vi "Connection Manager (customizable TDT).vi"(9 "Required":cluster{"DI":string[]}[](array[cluster]), 11 "Configuration file":path=path "C:/ProgramData/EPL/Tosca Defaults.ini") -> (2 "changed?":bool)   [LabVIEW 2020]
uses:
  Utility VIs/Controls/KTable/KTable.xctl
  Utility VIs/Controls/KListboxEx/KListboxEx.xctl
  PXI DAQ VIs/TDT VIs/Typedefs/TDT-Input source.ctl
  Type Defs/CM-Connection.ctl
  Utility VIs/Controls/KTable/Event Type.ctl
  PXI DAQ VIs/TDT VIs/TDT-Globals.vi
panel:
  in  "AI List":i32(xcontrol) caption="Inputs"
  in  "DI List":i32(xcontrol) caption="Inputs"
  in  "AO List":i32(xcontrol) caption="Outputs"
  in  "DO List":i32(xcontrol) caption="Outputs"
  in  "Apply Button":bool
  out "Save Op":enum16{"None", "Save", "Save and Exit"}(ring)
  in  "Exit":bool
  in  "DO Table":u16(xcontrol)
  out "show device":bool
  out "Image":enum32{"Blank", "RX6", "RZ5", "RZ6"}(tab)
  in  "Input source":u16(ring) items=["Front panel", "RA4LI", "RA16LI"]
  in  "Run on":i16(ring) items=[""=-1, "RX6"=0, "RZ5"=1, "RZ6"=2]
  in  "DI Table":u16(xcontrol)
  in  "AI Table":u16(xcontrol)
  out "read config":bool
  out "show connections":bool
  in  "AO Table":u16(xcontrol)
  # "ANALOG"
  # "DIGITAL"
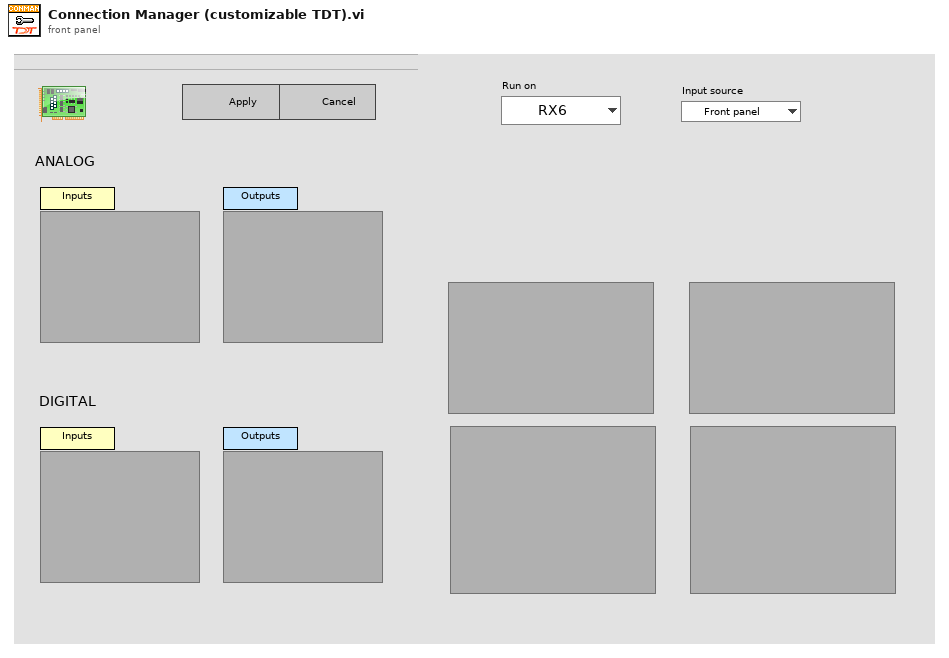
[diagram p1: front panel]
types:
  T1 = typedef "KListboxEx.xctl/Events.ctl" = cluster{"Items Changed":refnum<user-event>, "List Changed":refnum<user-event>}
  T2 = typedef "KTable.xctl/Events.ctl" = cluster{"Items Changed":refnum<user-event>}
  T3 = typedef "TDT-Input source.ctl" = enum16{"Front Panel", "RA4LI", "RA16LI"}
  T4 = typedef "KTable.xctl/Event Type.ctl" = enum16{"None", "Selection", "Edit", "Insert", "Delete", "Up", "Down", "Duplicate"}
  T5 = typedef "TDT-Output source.ctl" = cluster{"Device":T6, "Num":i32}
  T6 = typedef "TDT-Device ID.ctl" = enum16{"None", "PA5", "RP2", "RL2", "RA16", "RV8", "RX5", "RX6", "RX7", "RX8", "RZ2", "RZ5", "RZ6"}
  T7 = typedef "TDT-Device Config.ctl" = cluster{"Output":T5, "Input":T3}
  T8 = typedef "CM-Connection.ctl" = cluster{"IOChannel":string, "Endpoint":string}
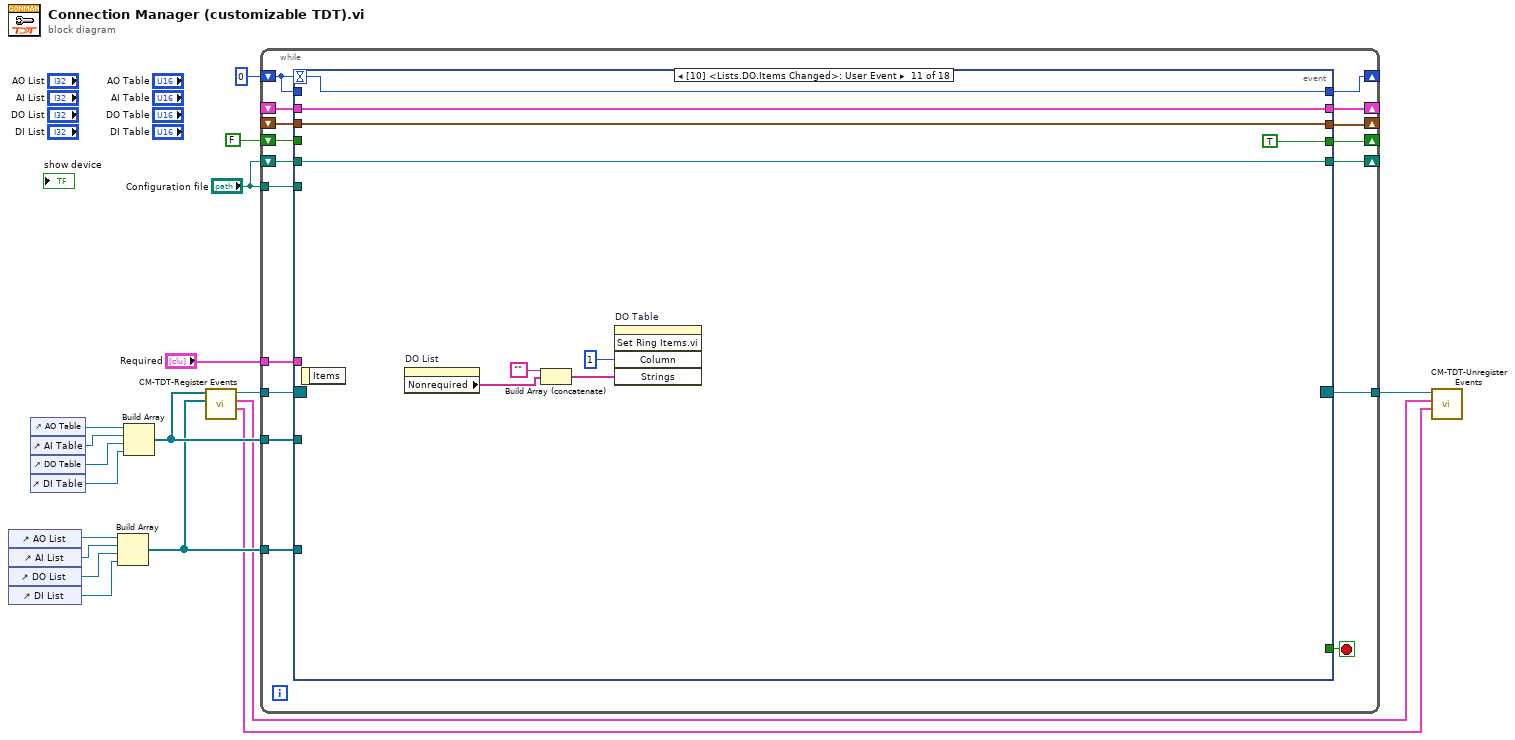
[diagram p0: block diagram]
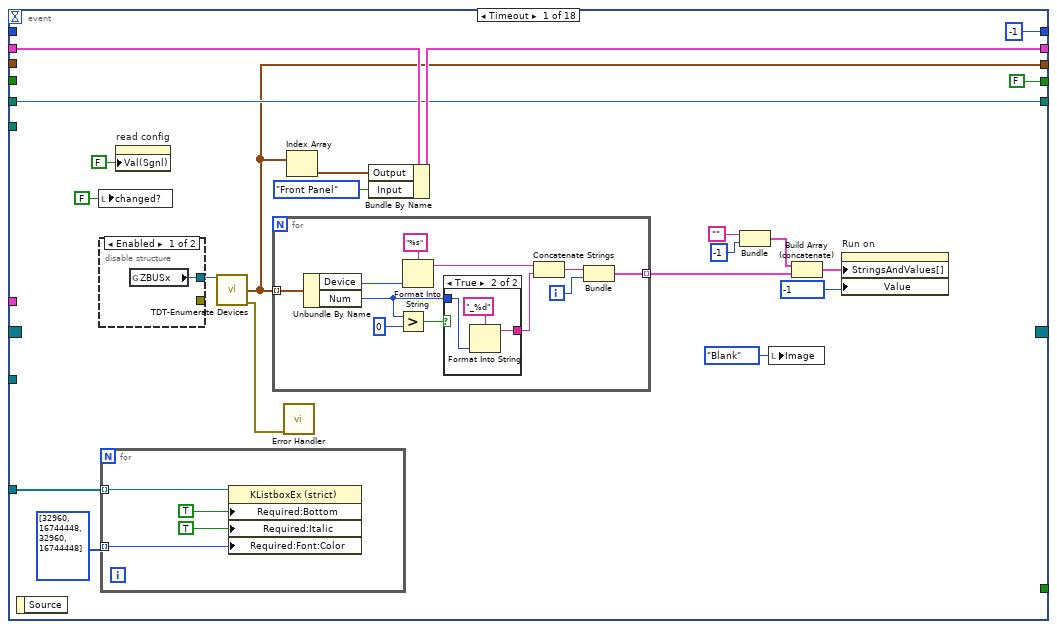
[diagram p2: hidden frame]
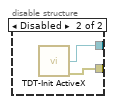
[diagram p3: hidden frame]
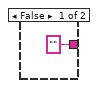
[diagram p4: hidden frame]
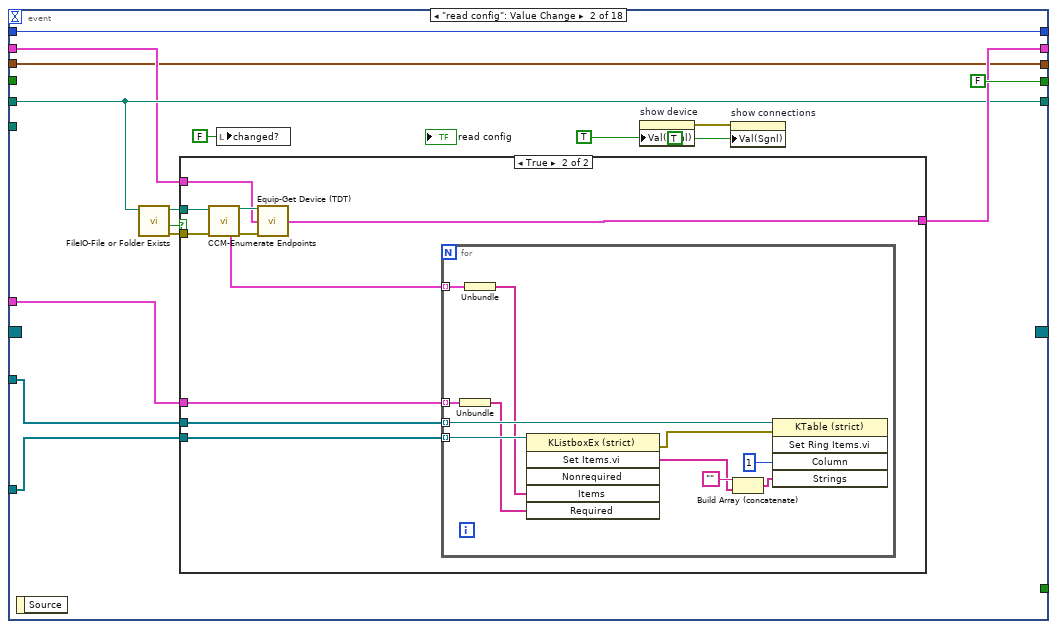
[diagram p5: hidden frame]
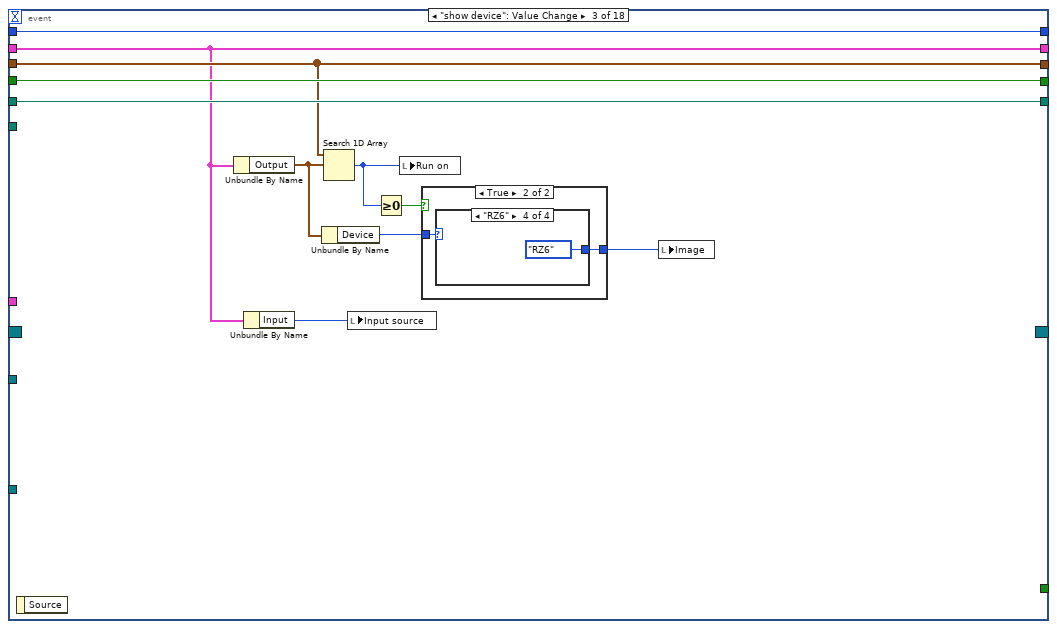
[diagram p7: hidden frame]
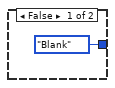
[diagram p8: hidden frame]
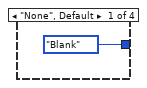
[diagram p9: hidden frame]
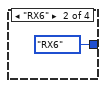
[diagram p10: hidden frame]
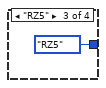
[diagram p11: hidden frame]
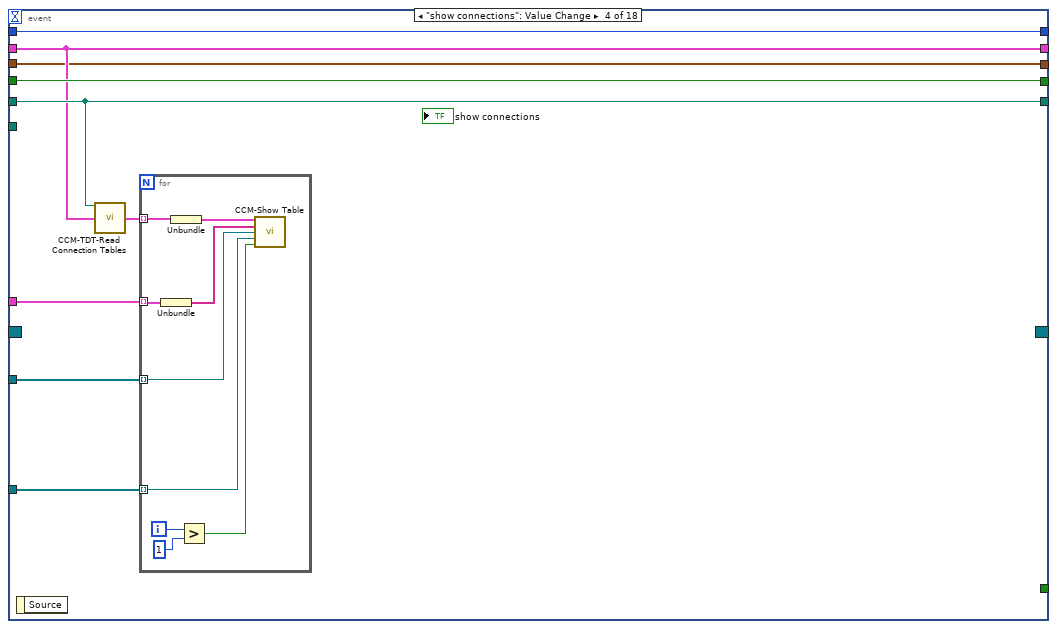
[diagram p12: hidden frame]
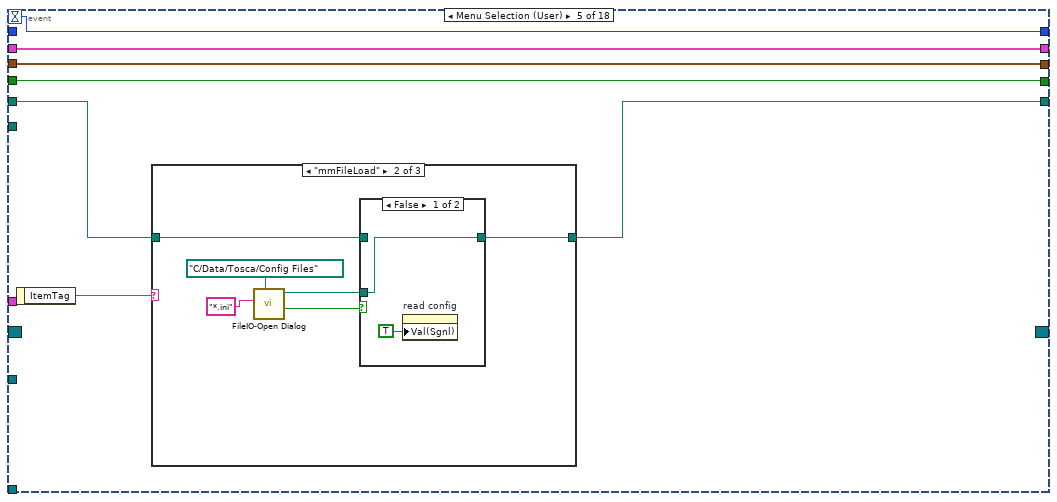
[diagram p13: hidden frame]
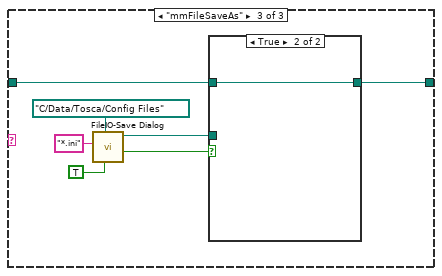
[diagram p16: hidden frame]
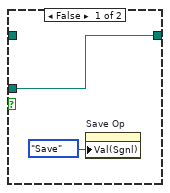
[diagram p17: hidden frame]
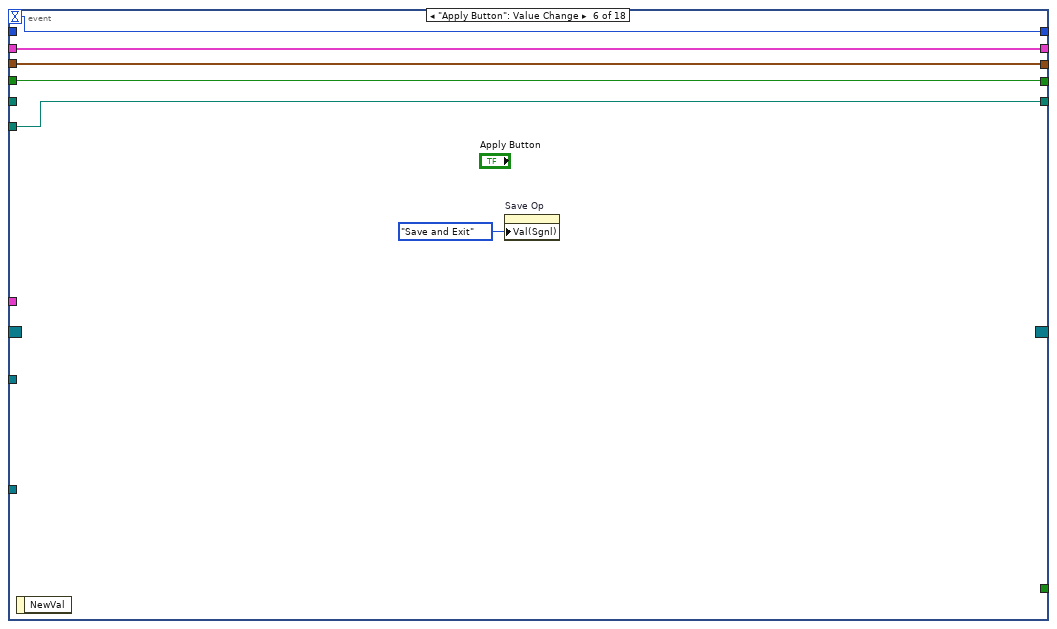
[diagram p18: hidden frame]
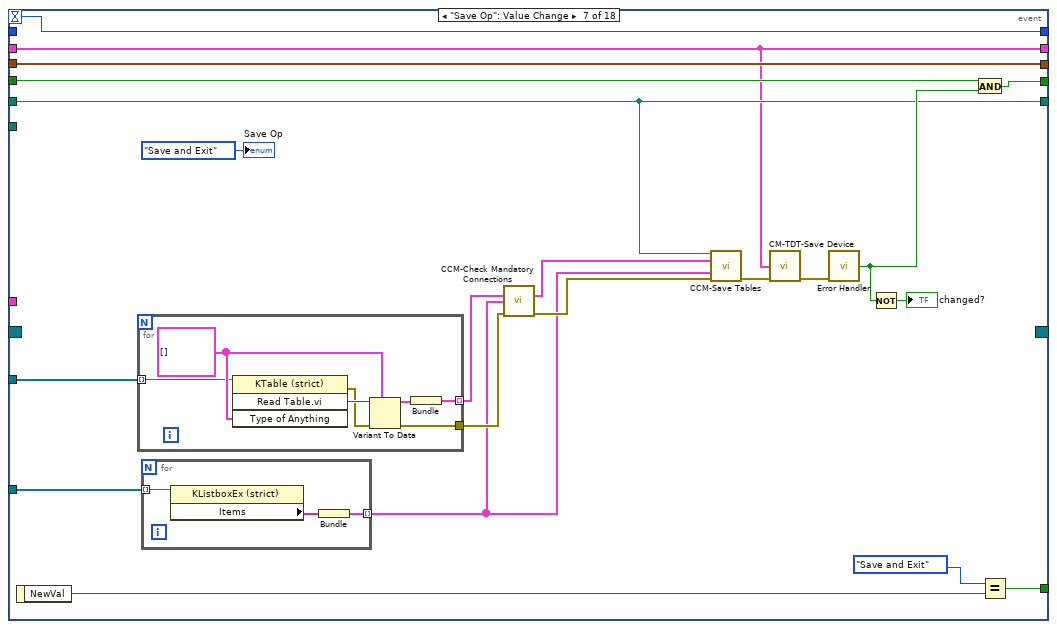
[diagram p19: hidden frame]
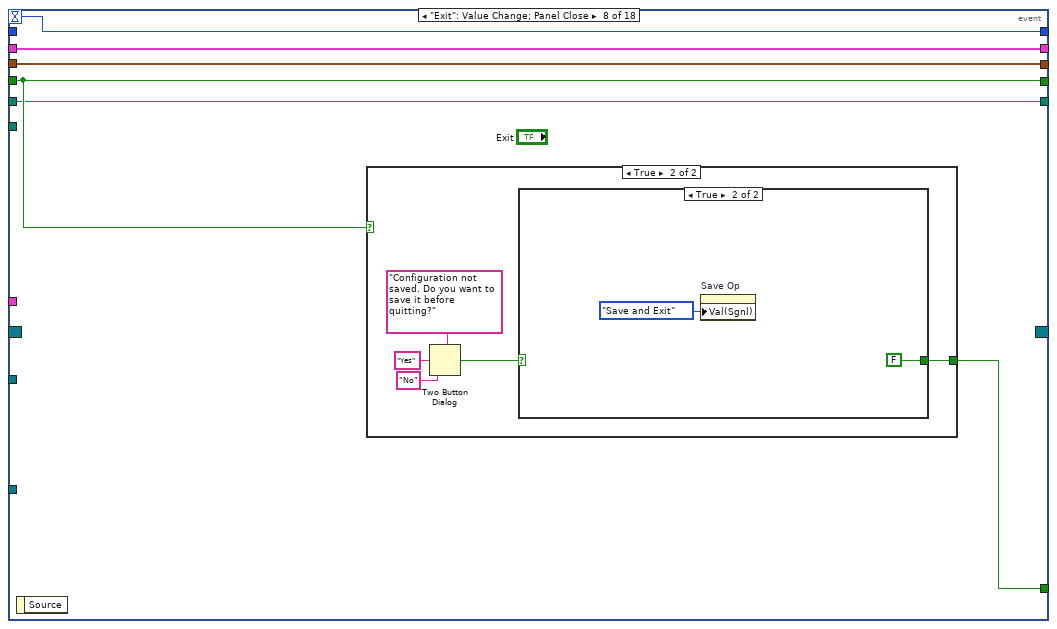
[diagram p20: hidden frame]
diagram:
  n1 = control-ref of="AO List"() -> (w6:refnum<vi>)
  n2 = control-ref of="AI List"() -> (w11:refnum<vi>)
  n3 = control-ref of="DO List"() -> (w10:refnum<vi>)
  n4 = control-ref of="DI List"() -> (w5:refnum<vi>)
  n5 = control-ref of="AO Table"() -> (w14:refnum<vi>)
  n6 = control-ref of="AI Table"() -> (w13:refnum<vi>)
  n7 = control-ref of="DO Table"() -> (w9:refnum<vi>)
  n8 = control-ref of="DI Table"() -> (w12:refnum<vi>)
  n9 = Build Array(w6, w11, w10, w5) -> (w7:refnum<vi>[])
  n10 = Build Array(w14, w13, w9, w12) -> (w8:refnum<vi>[])
  n11 = call "CM-TDT-Register Events.vi"("List Refs"=w7, "Table Refs"=w8) -> ("Lists"=w2:cluster{"AO":T1, "AI":T1, "DO":T1, "DI":T1}, "Tables"=w3:cluster{"AO":T2, "AI":T2, "DO":T2, "DI":T2}, "Event Registration Refnum"=w16:refnum<event-registration>)  [unwired: 7 in]
  n12 = while {
    shift-right: [w34] -> _
    shift-left: 0 -> [w29]
    shift-right: [w31] -> _
    shift-left: FALSE -> [w32]
    tunnel: "Required" -> [w30]
    tunnel: w16 -> [w28]
    shift-right: [w27] -> _
    shift-left: _ -> [w26]
    shift-right: [w25] -> _
    shift-left: "Configuration file" -> [w33]
    tunnel: "Configuration file" -> [w24]
    tunnel: w8 -> [w23]
    shift-right: [w22] -> _
    shift-left: _ -> [w21]
    tunnel: w7 -> [w20]
    tunnel: [w19] -> w4
    stop <- w35 stop-if-true
    n13 = event shown="[10] <Lists.DO.Items Changed>: User Event" {
      selector: w28 -> [_ _ _ _ _ _ _ _ _ _ _ _ _ _ _ _ _ _]
      dyn-events: [_ _ _ _ _ _ _ _ _ _ _ _ _ _ _ _ _ _] -> w19
      timeout: w29 -> [_ _ _ _ w159 w184 w206 w222 w240 w249 w258 w267 _ _ _ _ _ _]
      tunnel: [_ _ _ _ _ _ w202 w221 _ _ _ _ _ _ _ _ _ _] -> w35
      tunnel: [-1 w89 w127 w142 w159 w184 w206 w222 w240 w249 w258 w267 w278 w290 w299 w308 w317 w326] -> w34
      tunnel: w33 -> [w49 w87 w125 w141 w155 _ w197 w218 w238 w247 w256 w265 w276 w288 w297 w306 w315 w324]
      tunnel: w32 -> [_ _ w126 w143 w158 w183 w201 w220 _ _ _ _ _ _ w293 w302 w311 w320]
      tunnel: [FALSE FALSE w126 w143 w158 w183 w200 w220 TRUE TRUE TRUE TRUE TRUE TRUE w292 w301 w310 w319] -> w31
      tunnel: w30 -> [_ w79 _ w136 _ _ _ _ _ _ _ _ _ _ _ _ _ _]
      tunnel: w29 -> [_ w89 w127 w142 _ _ _ _ _ _ _ _ w278 w290 w299 w308 w317 w326]
      tunnel: [w51 w88 w121 w140 w156 w182 w189 w219 w239 w248 w257 w266 w275 w286 w298 w307 w316 w325] -> w27
      tunnel: w26 -> [w52 w86 w121 w140 w156 w182 w189 w219 w239 w248 w257 w266 w277 w289 w298 w307 w316 w325]
      tunnel: [w49 w87 w125 w141 w154 w181 w197 w218 w238 w247 w256 w265 w276 w288 w297 w306 w315 w324] -> w25
      tunnel: w24 -> [_ _ _ _ _ w181 _ _ _ _ _ _ _ _ _ _ _ _]
      tunnel: w23 -> [_ w85 _ w137 _ _ w194 _ _ _ _ _ _ _ _ _ _ _]
      tunnel: [w47 w84 w124 w139 w153 w180 w195 w217 w237 w246 w255 w264 w274 w287 w296 w305 w314 w323] -> w22
      tunnel: w21 -> [_ w84 w124 w139 w153 w180 w195 w217 w237 w246 w255 w264 w274 w287 w296 w305 w314 w323]
      tunnel: w20 -> [w37 w80 _ w135 _ _ w192 _ _ _ _ _ _ _ _ _ _ _]
      event Timeout {
        w40 = i16 -1 items=["", "RZ5_1"] ("Run on")
        n14 = event-data() -> ()  [unwired: 1 in, 1 out]
        n15 = local write "changed?"(FALSE ("changed?")) -> ()
        n16 = disable-structure shown="Enabled" {
          disable-tunnel: [w61 w63] -> w53
          disable-tunnel: [_ w62] -> _
          frame Enabled {
            n17 = global read "TDT-Globals.vi" "ZBUSx"() -> (w61:refnum<k7>)
          }
          frame Disabled {
            n18 = call "TDT-Init ActiveX.vi"() -> ("ZBUSx"=w63:refnum<k7>, "error out"=w62:errorcluster)  [unwired: 12 in, 2 out]
          }
        }
        n19 = for {
          tunnel: w37 -> [w58] mode=indexing
          tunnel: u32[] [32960, 16744448, 32960, 16744448] -> [w57] mode=indexing
          n20 = property class="KListboxEx (strict)"(reference=w58, "Required:Bottom"=TRUE, "Required:Italic"=TRUE ("Required:Font:Italic"), "Required:Font:Color"=w57) -> ()  [unwired: 1 in, 2 out]
        }
        n21 = property on="read config" class="Bool (strict)"("Val(Sgnl)"=FALSE ("Value (Signaling)")) -> ()  [unwired: 2 in, 2 out]
        n22 = call "TDT-Enumerate Devices.vi"("ZBUSx In"=w53) -> ("Devices"=w47:T5[], "error out"=w38:errorcluster)  [unwired: 12 in, 1 out]
        n23 = for {
          tunnel: w47 -> [w74] mode=indexing
          tunnel: [w65] -> w42 mode=indexing
          i -> [w64]
          n24 = Unbundle By Name(w74) -> ("Device"=w66:T6, "Num"=w69:i32)
          n25 = Greater?(x=w69, y=0) -> (0:w70:bool)
          n26 = Format Into String(format string="%s", w66) -> (resulting string=w72:string)  [unwired: 2 in, 1 out]
          n27 = case shown="True" w70 {
            tunnel: w69 -> [_ w77]
            tunnel: ["" w76] -> w67
            frame False {
            }
            frame True {
              n28 = Format Into String(format string="_%d", w77) -> (resulting string=w76:string)  [unwired: 2 in, 1 out]
            }
          }
          n29 = Concatenate Strings(w72, w67) -> (w68:string)
          n30 = Bundle(w68, w64) -> (w65:cluster{string, i32})  [unwired: 1 in]
        }
        n31 = call "Error Handler.vi"("error in (no error)"=w38) -> ()  [unwired: 13 in, 2 out]
        n32 = Index Array(array=w47) -> (element=w50:T5)  [unwired: 1 in]
        n33 = Bundle By Name(cluster=w52, "Output"=w50, "Input"=TDT-Input_source."Front Panel") -> (w51:T7)
        n34 = Bundle("", -1) -> (w41:cluster{string, i32})  [unwired: 1 in]
        n35 = local write "Image"(enum32{"Blank", "RX6", "RZ5"}."Blank" ("Image")) -> ()
        n36 = Build Array (concatenate)(w41, w42) -> (w43:cluster{string, i32}[])
        n37 = property on="Run on" class="Ring (strict)"("StringsAndValues[]"=w43, "Value"=w40) -> ()  [unwired: 2 in, 2 out]
      }
      event "read config": Value Change {
        n38 = event-data() -> ()  [unwired: 1 in, 1 out]
        n39 = call "FileIO-File or Folder Exists.vi"("path"=w87) -> ("error out"=w93:errorcluster, "Exists?"=w92:bool, "dup path"=w94:path)  [unwired: 7 in, 1 out]
        n40 = case shown="True" w92 {
          tunnel: w94 -> [_ w105]
          tunnel: w93 -> [_ w104]
          tunnel: [w95 w100] -> w88
          tunnel: w86 -> [w95 w101]
          tunnel: w85 -> [_ w99]
          tunnel: w80 -> [_ w98]
          tunnel: w79 -> [_ w97]
          frame False {
          }
          frame True {
            n41 = call "CCM-Enumerate Endpoints.vi"("Path In"=w105, "error in (no error)"=w104) -> ("Path Out"=w102:path, "Endpoints"=w96:cluster{"Name":string[]}[], "error out"=w103:errorcluster)  [unwired: 9 in, 2 out]
            n42 = call "Equip-Get Device (TDT).vi"("Path In"=w102, "Default"=w101, "error in (no error)"=w103) -> ("TDT-Device Config"=w100:T7)  [unwired: 10 in, 2 out]
            n43 = for {
              tunnel: w99 -> [w113] mode=indexing
              tunnel: w98 -> [w112] mode=indexing
              tunnel: w96 -> [w110] mode=indexing
              tunnel: w97 -> [w109] mode=indexing
              n44 = Unbundle(w109) -> ("DI"=w108:string[])
              n45 = Unbundle(w110) -> ("Name"=w107:string[])
              n46 = invoke on="Invoke Node" class="KListboxEx (strict)" method="Set Items.vi"(reference=w112, "Items"=w107, "Required"=w108) -> (error out=w111:errorcluster, "Set Items.vi"=w106:string[])  [unwired: 3 in, 4 out]
              n47 = Build Array (concatenate)("", w106) -> (w115:string[])
              n48 = invoke on="Invoke Node" class="KTable (strict)" method="Set Ring Items.vi"(reference=w113, error in=w111, "Column"=1, "Strings"=w115) -> ()  [unwired: 1 in, 5 out]
            }
          }
        }
        n49 = local write "changed?"(FALSE ("changed?")) -> ()
        n50 = property on="show device" class="Bool (strict)"("Val(Sgnl)"=TRUE ("Value (Signaling)")) -> (error out=w82:errorcluster)  [unwired: 2 in, 1 out]
        n51 = property on="show connections" class="Bool (strict)"(error in=w82, "Val(Sgnl)"=TRUE ("Value (Signaling)")) -> ()  [unwired: 1 in, 2 out]
      }
      event "show device": Value Change {
        n52 = event-data() -> ()  [unwired: 1 in, 1 out]
        n53 = Unbundle By Name(w121) -> ("Output"=w122:T5)
        n54 = Unbundle By Name(w121) -> ("Input"=w120:T3)
        n55 = Unbundle By Name(w122) -> ("Device"=w123:T6)
        n56 = Search 1D Array(1D array=w124, element=w122) -> (index of element=w119:i32)  [unwired: 1 in]
        n57 = local write "Input source"(w120) -> ()
        n58 = Greater Or Equal To 0?(x=w119) -> (x >= 0?=w118:bool)
        n59 = local write "Run on"(w119) -> ()
        n60 = case shown="True" w118 {
          tunnel: w123 -> [_ w130]
          tunnel: [enum32{"Blank", "RX6", "RZ5"}."Blank" ("Image") w129] -> w117
          frame False {
          }
          frame True {
            n61 = case shown="\"RZ6\"" w130 {
              tunnel: [enum32{"Blank", "RX6", "RZ5"}."Blank" ("Image") enum32{"Blank", "RX6", "RZ5"}."RX6" ("Image") enum32{"Blank", "RX6", "RZ5"}."RZ5" ("Image") enum32{"Blank", "RX6", "RZ5", "RZ6"}."RZ6" ("Image")] -> w129
              frame "None", Default {
              }
              frame "RX6" {
              }
              frame "RZ5" {
              }
              frame "RZ6" {
              }
            }
          }
        }
        n62 = local write "Image"(w117) -> ()
      }
      event "show connections": Value Change {
        n63 = event-data() -> ()  [unwired: 1 in, 1 out]
        n64 = call "CCM-TDT-Read Connection Tables.vi"("Path In"=w141, "TDT-Device Config"=w140) -> ("Tables"=w138:cluster{"Table":T8[]}[])  [unwired: 12 in, 1 out]
        n65 = for {
          tunnel: w138 -> [w150] mode=indexing
          tunnel: w137 -> [w146] mode=indexing
          tunnel: w136 -> [w148] mode=indexing
          tunnel: w135 -> [w145] mode=indexing
          i -> [w152]
          n66 = Unbundle(w148) -> ("DI"=w147:string[])
          n67 = Unbundle(w150) -> ("Table"=w149:T8[])
          n68 = Greater?(x=w152, y=1) -> (0:w144:bool)
          n69 = call "CCM-Show Table.vi"("Table"=w149, "Required"=w147, "Table Ref"=w146, "List Ref"=w145, "Force required"=w144) -> ()  [unwired: 11 in]
        }
      }
      event Menu Selection (User) {
        n70 = event-data() -> ("ItemTag"=w157:string)  [unwired: 1 in]
        n71 = case shown="\"mmFileLoad\"" w157 {
          tunnel: w155 -> [w160 w162 w171]
          tunnel: [w160 w161 w170] -> w154
          frame "False", Default {
          }
          frame "mmFileLoad" {
            n72 = call "FileIO-Open Dialog.vi"("Default Folder"=path "C:/Data/Tosca/Config Files", "pattern (all files)"="*.ini") -> ("cancelled"=w164:bool, "selected path"=w163:path)  [unwired: 7 in, 1 out]
            n73 = case shown="False" w164 {
              tunnel: w163 -> [w168 _]
              tunnel: w162 -> [_ w169]
              tunnel: [w168 w169] -> w161
              frame False {
                n74 = property on="read config" class="Bool (strict)"("Val(Sgnl)"=TRUE ("Value (Signaling)")) -> ()  [unwired: 2 in, 2 out]
              }
              frame True {
              }
            }
          }
          frame "mmFileSaveAs" {
            n75 = call "FileIO-Save Dialog.vi"("Overwrite prompt?"=TRUE, "Default Folder"=path "C:/Data/Tosca/Config Files", "pattern (all files)"="*.ini") -> ("cancelled"=w173:bool, "selected path"=w172:path)  [unwired: 6 in, 1 out]
            n76 = case shown="True" w173 {
              tunnel: w172 -> [w177 _]
              tunnel: w171 -> [_ w179]
              tunnel: [w177 w179] -> w170
              frame False {
                n77 = property on="Save Op" class="Enum (strict)"("Val(Sgnl)"=enum16{"None", "Save", "Save and Exit"}."Save" ("Value (Signaling)")) -> ()  [unwired: 2 in, 2 out]
              }
              frame True {
              }
            }
          }
        }
      }
      event "Apply Button": Value Change {
        n78 = event-data() -> ()  [unwired: 1 in, 1 out]
        n79 = property on="Save Op" class="Enum (strict)"("Val(Sgnl)"=enum16{"None", "Save", "Save and Exit"}."Save and Exit" ("Value (Signaling)")) -> ()  [unwired: 2 in, 2 out]
      }
      event "Save Op": Value Change {
        n80 = event-data() -> ("NewVal"=w204:enum16{"None", "Save", "Save and Exit"})  [unwired: 1 in]
        n81 = for {
          tunnel: [w211] -> w188 mode=indexing
          tunnel: w194 -> [w210] mode=indexing
          tunnel: [w214] -> w193
          w213 = T8[] []
          n82 = invoke on="Invoke Node" class="KTable (strict)" method="Read Table.vi"(reference=w210, "Type of Anything"=w213) -> (error out=w215:errorcluster, "Read Table.vi"=w216:variant)  [unwired: 2 in, 2 out]
          n83 = Variant To Data(error in=w215, type=w213, Variant=w216) -> (data=w212:T8[], error out=w214:errorcluster)
          n84 = Bundle(w212) -> (w211:cluster{T8[]})  [unwired: 1 in]
        }
        n85 = for {
          tunnel: w192 -> [w209] mode=indexing
          tunnel: [w207] -> w186 mode=indexing
          n86 = property class="KListboxEx (strict)"(reference=w209) -> ("Items"=w208:string[])  [unwired: 1 in, 2 out]
          n87 = Bundle("Items"=w208) -> (w207:cluster{"Items":string[]})  [unwired: 1 in]
        }
        n88 = call "CCM-Check Mandatory Connections.vi"("Tables"=w188, "Mandatory"=w186, "error in (no error)"=w193) -> ("Tables thru"=w187:cluster{"Table":T8[]}[], "error out"=w196:errorcluster)  [unwired: 11 in]
        n89 = call "CCM-Save Tables.vi"("configuration file path"=w197, "Tables"=w187, "Endpoints"=w186, "error in (no error)"=w196) -> ("error out"=w191:errorcluster)  [unwired: 10 in, 1 out]
        n90 = call "CM-TDT-Save Device.vi"("Device"=w189, "error in (no error)"=w191) -> ("error out"=w190:errorcluster)  [unwired: 13 in]
        n91 = call "Error Handler.vi"("error in (no error)"=w190) -> ("error?"=w199:bool)  [unwired: 13 in, 1 out]
        n92 = Not(x=w199) -> (.not. x?=→"changed?":bool)
        n93 = And(x=w201, y=w199) -> (x .and. y?=w200:bool)
        n94 = Equal?(x=enum16{"None", "Save", "Save and Exit"}."Save and Exit", y=w204) -> (x = y?=w202:bool)
        "Save Op" <- enum16{"None", "Save", "Save and Exit"}."Save and Exit" ("Save Op")
      }
      event "Exit": Value Change; Panel Close {
        n95 = event-data() -> ()  [unwired: 1 in, 1 out]
        n96 = case shown="True" w220 {
          tunnel: [TRUE w224] -> w221
          frame False {
          }
          frame True {
            n97 = Two Button Dialog(message="Configuration not saved. Do you want to save it before quitting?", 1:"No" ("F button name (\"Cancel\")"), 2:"Yes" ("T button name (\"OK\")")) -> (T button?=w225:bool)
            n98 = case shown="True" w225 {
              tunnel: [TRUE FALSE] -> w224
              frame False {
              }
              frame True {
                n99 = property on="Save Op" class="Enum (strict)"("Val(Sgnl)"=enum16{"None", "Save", "Save and Exit"}."Save and Exit" ("Value (Signaling)")) -> ()  [unwired: 2 in, 2 out]
              }
            }
          }
        }
      }
      event User Event {
        n100 = event-data() -> ("Items"=w232:string[])  [unwired: 1 in]
        n101 = Build Array (concatenate)("", w232) -> (w235:string[])
        n102 = invoke on="AO Table" class="KTable (strict)" method="Set Ring Items.vi"("Column"=1, "Strings"=w235) -> ()  [unwired: 3 in, 5 out]
      }
      event User Event {
        n103 = event-data() -> ("Items"=w241:string[])  [unwired: 1 in]
        n104 = Build Array (concatenate)("", w241) -> (w244:string[])
        n105 = invoke on="AI Table" class="KTable (strict)" method="Set Ring Items.vi"("Column"=1, "Strings"=w244) -> ()  [unwired: 3 in, 5 out]
      }
      event User Event {
        n106 = event-data() -> ()  [unwired: 1 in, 1 out]
        n107 = property on="DO List" class="KListboxEx (strict)"() -> ("Nonrequired"=w250:string[])  [unwired: 2 in, 2 out]
        n108 = Build Array (concatenate)("", w250) -> (w253:string[])
        n109 = invoke on="DO Table" class="KTable (strict)" method="Set Ring Items.vi"("Column"=1, "Strings"=w253) -> ()  [unwired: 3 in, 5 out]
      }
      event User Event {
        n110 = event-data() -> ()  [unwired: 1 in, 1 out]
        n111 = property on="DI List" class="KListboxEx (strict)"() -> ("Nonrequired"=w259:string[])  [unwired: 2 in, 2 out]
        n112 = Build Array (concatenate)("", w259) -> (w262:string[])
        n113 = invoke on="DI Table" class="KTable (strict)" method="Set Ring Items.vi"("Column"=1, "Strings"=w262) -> ()  [unwired: 3 in, 5 out]
      }
      event "Run on": Value Change {
        n114 = event-data() -> ()  [unwired: 1 in, 1 out]
        n115 = Index Array(array=w274, index="Run on") -> (element=w272:T5)
        n116 = Unbundle By Name(w272) -> ("Device"=w271:T6)
        n117 = Bundle By Name(cluster=w277, "Output"=w272) -> (w275:T7)
        n118 = case shown="\"RZ6\"" w271 {
          tunnel: [enum32{"Blank", "RX6", "RZ5"}."Blank" ("Image") enum32{"Blank", "RX6", "RZ5"}."RX6" ("Image") enum32{"Blank", "RX6", "RZ5"}."RZ5" ("Image") enum32{"Blank", "RX6", "RZ5", "RZ6"}."RZ6" ("Image")] -> w268
          frame "None", Default {
          }
          frame "RX6" {
          }
          frame "RZ5" {
          }
          frame "RZ6" {
          }
        }
        "Image" <- w268
        n119 = property on="show connections" class="Bool (strict)"("Val(Sgnl)"=TRUE ("Value (Signaling)")) -> ()  [unwired: 2 in, 2 out]
      }
      event "Input source": Value Change {
        n120 = event-data() -> ()  [unwired: 1 in, 1 out]
        n121 = Bundle By Name(cluster=w289, "Input"="Input source") -> (w286:T7)
        n122 = property on="show connections" class="Bool (strict)"("Val(Sgnl)"=TRUE ("Value (Signaling)")) -> ()  [unwired: 2 in, 2 out]
      }
      event User Event {
        n123 = event-data() -> ("Type"=w291:T4)  [unwired: 1 in]
        n124 = Equal?(x=w291, y=Event_Type."Edit") -> (x = y?=w294:bool)
        n125 = Or(x=w293, y=w294) -> (x .or. y?=w292:bool)
      }
      event User Event {
        n126 = event-data() -> ("Type"=w300:T4)  [unwired: 1 in]
        n127 = Equal?(x=w300, y=Event_Type."Edit") -> (x = y?=w303:bool)
        n128 = Or(x=w302, y=w303) -> (x .or. y?=w301:bool)
      }
      event User Event {
        n129 = event-data() -> ("Type"=w309:T4)  [unwired: 1 in]
        n130 = Equal?(x=w309, y=Event_Type."Edit") -> (x = y?=w312:bool)
        n131 = Or(x=w311, y=w312) -> (x .or. y?=w310:bool)
      }
      event User Event {
        n132 = event-data() -> ("Type"=w318:T4)  [unwired: 1 in]
        n133 = Equal?(x=w318, y=Event_Type."Edit") -> (x = y?=w321:bool)
        n134 = Or(x=w320, y=w321) -> (x .or. y?=w319:bool)
      }
    }
  }
  n135 = call "CM-TDT-Unregister Events.vi"("Lists"=w2, "Tables"=w3, "Event Registration Refnum"=w4) -> ()  [unwired: 9 in]
